vi "ReactionTimer.vi"() -> ()   [LabVIEW 2014]
panel:
  in  "Stop timer":bool
  out "Waveform Chart 2":u32(graph)
  out "Reaction Time(ms)":u32
  in  "LED":bool
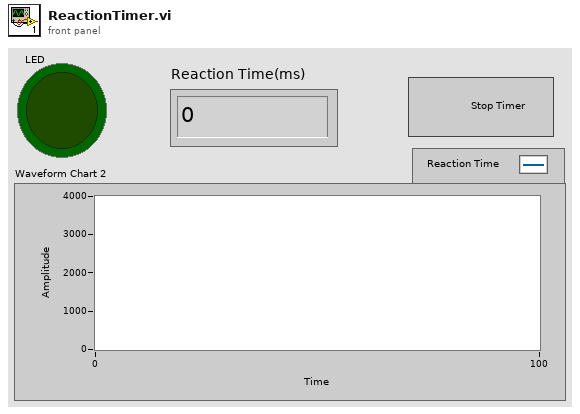
[diagram p1: front panel]
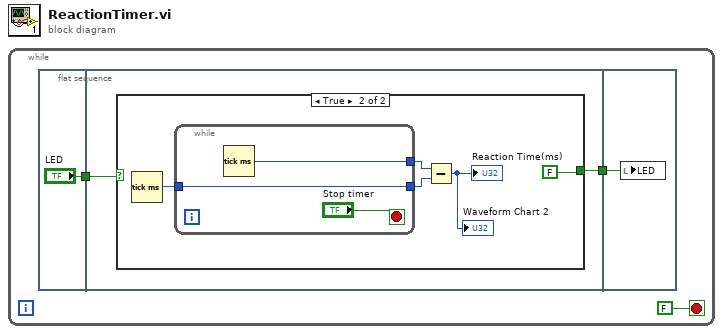
[diagram p0: block diagram]
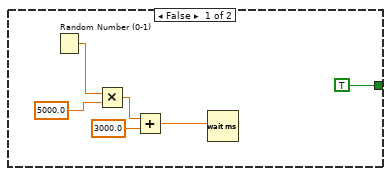
[diagram p2: hidden frame]
diagram:
  n1 = while {
    stop <- FALSE stop-if-true
    n2 = flat-sequence {
      tunnel: ["LED"] -> w3
      tunnel: w3 -> [w6]
      tunnel: [w5] -> w2
      tunnel: w2 -> [w21]
      frame #0 {
      }
      frame #1 {
        n3 = case shown="True" w6 {
          tunnel: [TRUE FALSE] -> w5
          frame False {
            n4 = Random Number (0-1)() -> (number: 0 to 1=w12:dbl)
            n5 = Multiply(x=w12, y=5000.0) -> (x*y=w10:dbl)
            n6 = Add(x=w10, y=3000.0) -> (x+y=w8:dbl)
            n7 = Wait (ms)(milliseconds to wait=w8) -> ()  [unwired: 1 out]
          }
          frame True {
            n8 = Tick Count (ms)() -> (millisecond timer value=w17:u32)
            n9 = while {
              tunnel: w17 -> [w19]
              tunnel: [w20] -> w16
              tunnel: [w19] -> w15
              stop <- "Stop timer" stop-if-true
              n10 = Tick Count (ms)() -> (millisecond timer value=w20:u32)
            }
            n11 = Subtract(x=w16, y=w15) -> (x-y=→"Reaction Time(ms)" →"Waveform Chart 2":u32)
          }
        }
      }
      frame #2 {
        n12 = local write "LED"(w21) -> ()
      }
    }
  }
